vi "QT_DynCall.vi"(0 "QT Ref In":T11, 1 "Frame Grabber Settings":T15={"Name"="", "Digitizer"=0, "Input"=0, "Witdh"=0, "Height"=0, "Input format"=enum."PAL", "Frame rate"=0.0, "Reserved"=0, "Dialogs"=0} {"Frame rate" format="%#1_6g"; "Dialogs" format="%.0b"}, 3 "Compression Settings":T14 {"Dialogs" format="%.0b"; "Comp. Quality" format="%.0x"; "Codec" format="%.0x"}, 4 "Movie Settings":T10 {"Dialogs" format="%.0b"}, 5 "Image in":T5 {"Dialogs" format="%.0b"}, 6 "Sound in":T4 {"Rate" format="%x"}, 7 "error in (no error)":errorcluster, 8 "Selector":T16=enum."Get QT & CIN info", 9 "Video Settings in":T3={"Color format"=1, "Hue"=0.0, "Saturation"=0.0, "Brightness"=0.0, "Contrast"=0.0, "Sharpness"=0.0, "Black Level"=0.0, "White Level"=0.0, "Options"=0, "Dialogs"=0} {"Dialogs" format="%.0b"; "Color format" items=["Black & White (8 bits)", "RGB (24 bits)", "RGBx (32 bits)", "RGBA (32bits)", "RGB B&W (32 bits)", "HSI (24 bits)", "HSIx (32 bits)", "HSI B&W (32 bits)"]; "Brightness" format="%.2f"; "Contrast" format="%.2f"; "Sharpness" format="%.2f"; "Black Level" format="%.2f"; "White Level" format="%.2f"; "Saturation" format="%.2f"; "Hue" format="%.2f"}, 12 "Private":T6={"reserved 1"=4, "reserved 2"=0, "reserved 3"=0, "reserved 4"=0}, 13 "Effect":T9 {"Matrix" format="%.2f"}, 15 "File Settings":T13 {"Dialogs" format="%.0b"}) -> (16 "Info Out":T12, 17 "Video Settings out":T3={"Color format"=1, "Hue"=0.0, "Saturation"=0.0, "Brightness"=0.0, "Contrast"=0.0, "Sharpness"=0.0, "Black Level"=0.0, "White Level"=0.0, "Options"=0, "Dialogs"=0} {"Dialogs" format="%.0b"; "Color format" items=["Black & White (8 bits)", "RGB (24 bits)", "RGBx (32 bits)", "RGBA (32bits)", "RGB B&W (32 bits)", "HSI (24 bits)", "HSIx (32 bits)", "HSI B&W (32 bits)"]; "Brightness" format="%.2f"; "Contrast" format="%.2f"; "Sharpness" format="%.2f"; "Black Level" format="%.2f"; "White Level" format="%.2f"; "Saturation" format="%.2f"; "Hue" format="%.2f"}, 20 "QT Ref Out":T11, 23 "Movie info":T7 {"Tracks"."Rate" format="%.2f"}, 24 "QT Info":T1 {"Digitizers"."In Flags" format="%.0b"; "Digitizers"."Out Flags" format="%.0b"; "Digitizers"."Inputs" items=["Composite", "S-Video", "RGB", "RGB Synch", "YUV", "YUV Synch", "TV Tuner", "sdiln"]; "CIN rev ID" format="%.2f"}, 25 "Image/Movie Out":T5 {"Dialogs" format="%.0b"}, 26 "Sound out":T4 {"Rate" format="%x"}, 27 "error out":errorcluster={"status"=TRUE, "code"=-43, "source"=""})   [LabVIEW 2009]
uses:
  QT_Selector.ctl
  QT_FrameGrabber.ctl
  QT_Video.ctl
  QT_Compression.ctl
  QT_File.ctl
  QT_ErrInfo.ctl
  QT_Image.ctl
  QT_Ref.ctl
  QT_Movie.ctl
  QT_Effect.ctl
  QT_MovieInfo.ctl
  QT_Track.ctl
  QT_Private.ctl
  QT_Sound.ctl
  QT_Info.ctl
  QT_Digitizer.ctl
panel:
  in  "type specifier VI Refnum (for type only)":refnum<vi>
  # "[0,0] [0,1]  [0,2] [1,0].. [2,2]"
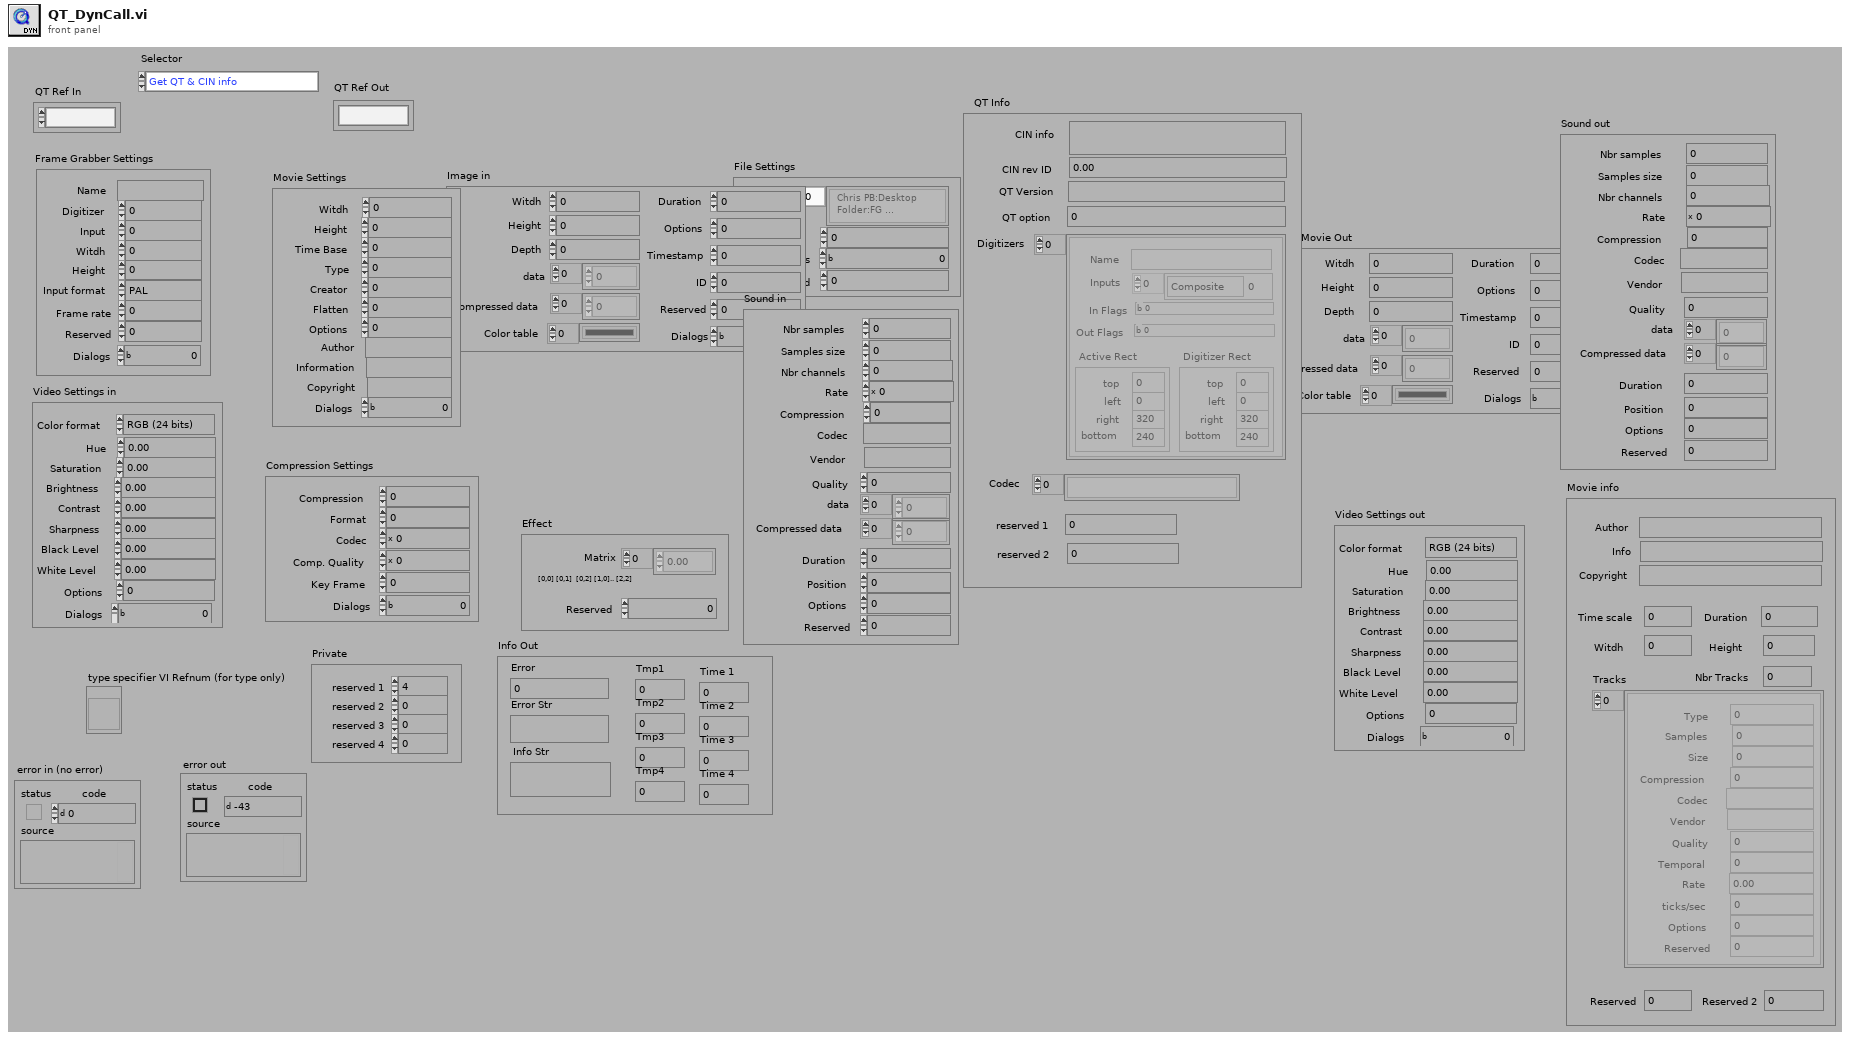
[diagram p1: front panel]
types:
  T1 = typedef "QT_Info.ctl" = cluster{"CIN info":string, "CIN rev ID":dbl, "QT Version":string, "QT option":i32, "Digitizers\n":T2[], "Codec":string[], "reserved 1":i32, "reserved 2":i32}
  T2 = typedef "QT_Digitizer.ctl" = cluster{"Name":string, "Inputs":i32[], "In Flags":i32, "Out Flags":i32, "Digitizer Rect":cluster{"top":i32, "left":i32, "right":i32, "bottom":i32}, "Active Rect":cluster{"top":i32, "left":i32, "right":i32, "bottom":i32}}
  T3 = typedef "QT_Video.ctl" = cluster{"Color format":u32, "Hue":dbl, "Saturation":dbl, "Brightness":dbl, "Contrast":dbl, "Sharpness":dbl, "Black Level":dbl, "White Level":dbl, "Options":i32, "Dialogs":u32}
  T4 = typedef "QT_Sound.ctl" = cluster{"Nbr samples":i32, "Samples size":i32, "Nbr channels":i32, "Rate ":i32, "Compression":i32, "Codec":string, "Vendor":string, "Quality":i32, "data":i16[], "Compressed data":u8[], "Duration":i32, "Position":i32, "Options":i32, "Reserved":i32}
  T5 = typedef "QT_Image.ctl" = cluster{"Witdh":i32, "Height":i32, "Depth":i32, "data":u8[], "Compressed data":u8[], "Color table":u32[], "Duration":i32, "Options":i32, "Timestamp":i32, "ID":i32, "Reserved":i32, "Dialogs":u32}
  T6 = typedef "QT_Private.ctl" = cluster{"reserved 1":i32, "reserved 2":i32, "reserved 3":i32, "reserved 4":i32}
  T7 = typedef "QT_MovieInfo.ctl" = cluster{"Author":string, "Info":string, "Copyright":string, "Time scale":i32, "Duration":i32, "Witdh":i32, "Height":i32, "Nbr Tracks":i32, "Tracks":T8[], "Reserved":i32, "Reserved 2":i32}
  T8 = typedef "QT_Track.ctl" = cluster{"Type":i32, "Samples":i32, "Size":i32, "Compression":i32, "Codec":string, "Vendor":string, "Quality":i32, "Temporal":i32, "Rate ":dbl, "ticks/sec":i32, "Options":i32, "Reserved":i32}
  T9 = typedef "QT_Effect.ctl" = cluster{"Reserved":i32, "Matrix":dbl[]}
  T10 = typedef "QT_Movie.ctl" = cluster{"Witdh":i32, "Height":i32, "Time Base":i32, "Type":i32, "Creator":i32, "Flatten":i32, "Options":i32, "Author":string, "Information":string, "Copyright":string, "Dialogs":u32}
  T11 = typedef "QT_Ref.ctl" = refnum<k1>
  T12 = typedef "QT_ErrInfo.ctl" = cluster{"Error":i32, "Error Str":string, "Info Str":string, "Tmp1":i32, "Tmp2":i32, "Tmp3":i32, "Tmp4":i32, "Time 1":i32, "Time 2":i32, "Time 3":i32, "Time 4":i32}
  T13 = typedef "QT_File.ctl" = cluster{"Paths":string[], "Options":i32, "Dialogs":u32, "Reserved":i32}
  T14 = typedef "QT_Compression.ctl" = cluster{"Compression":i32, "Format":i32, "Codec":i32, "Comp. Quality":i32, "Key Frame":i32, "Dialogs":u32}
  T15 = typedef "QT_FrameGrabber.ctl" = cluster{"Name":string, "Digitizer":i32, "Input":i32, "Witdh":i32, "Height":i32, "Input format":enum32{"NTSC", "PAL", "Secam"}, "Frame rate":dbl, "Reserved":i32, "Dialogs":u32}
  T16 = typedef "QT_Selector.ctl" = enum32{"do nothing", "Get all Sources", "Get Source info", "Open Image", "Save Image to File", "Effect", "Close", "SG Grab", "Compress in Memory", "Decompress to Memory", "New Movie", "Open Movie", "Add Frame", "Get Frame", "Close Movie", "Get QT & CIN info", "SG init", "SG Close", "Open sound file", "Close sound file", "Read sound data", "Write sound data", "Import sound", "Export sound", "Add sound to movie", "Get sound from movie", "reserved", "reserved 1", "reserved 2"}
  T17 = enum32{"invalid CPU target", "Motorola 68K", "PowerPC", "Intel x86", "SPARC", "PA-RISC", "MIPS", "Alpha"}
  T18 = enum32{"invalid OS target", "Mac OS", "Windows 3.1", "Windows 95/NT", "Solaris 1", "Solaris 2", "HP-UX", "PowerMAX", "Linux", "Irix", "Rhapsody", "BeOS", "AIX", "OSF1", "VxWorks", "PharLap", "Carbon", "RTX", "Windows x64", "Linux x64"}
  T19 = enum32{"invalid CPU target", "Motorola 68K", "PowerPC", "Intel x86", "SPARC", "PA-RISC", "MIPS", "Alpha", "ARM", "AMD/Intel x64"}
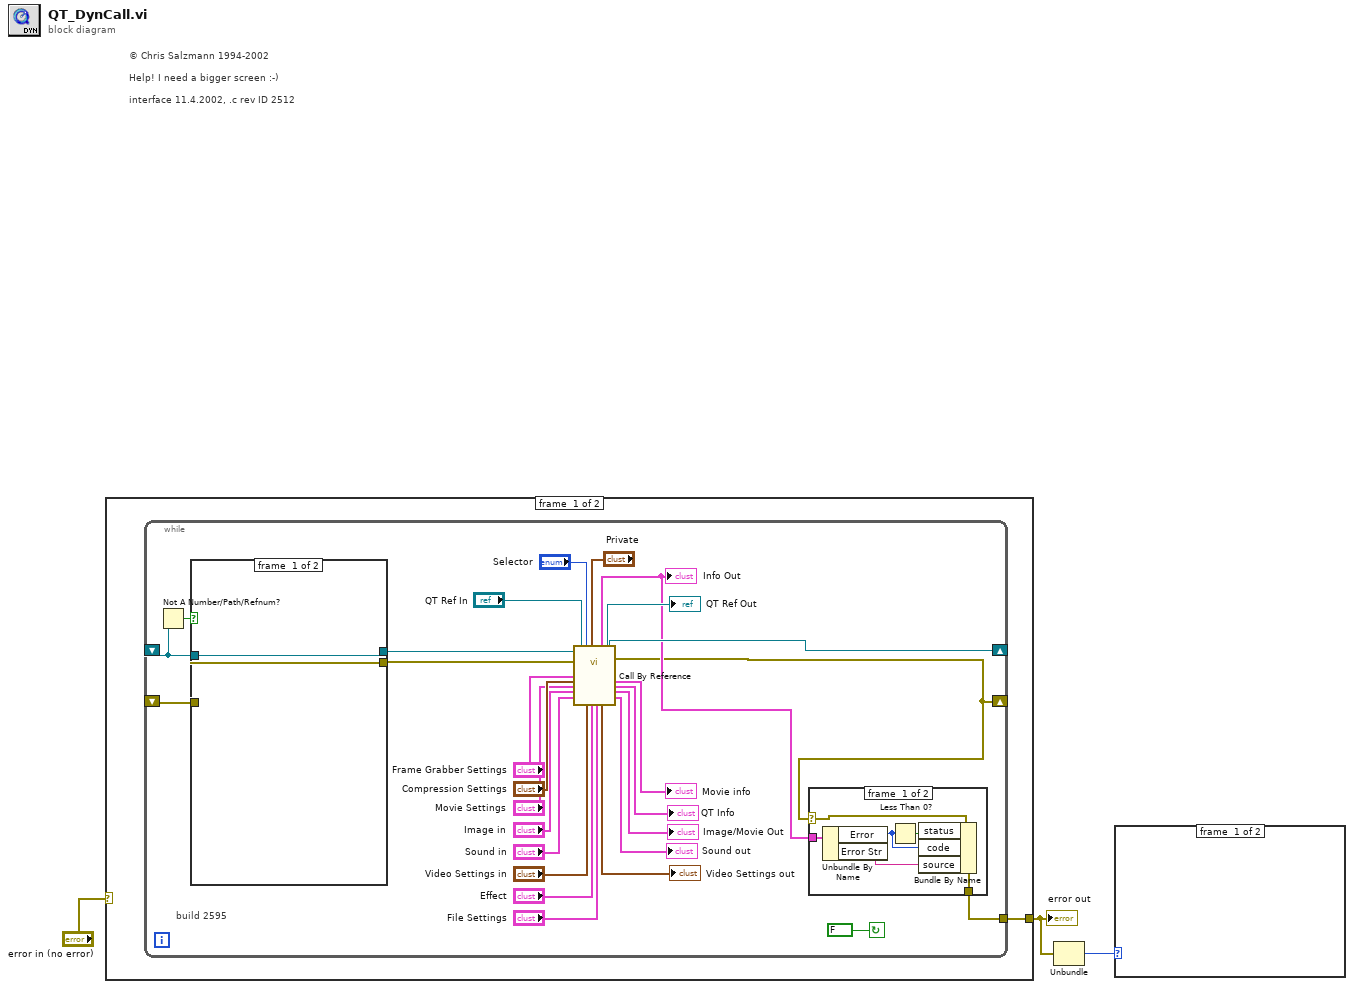
[diagram p0: block diagram]
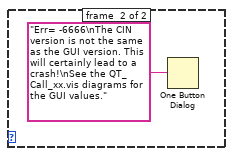
[diagram p2: hidden frame]
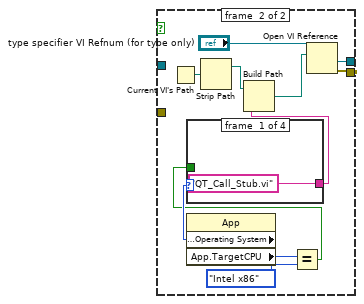
[diagram p4: hidden frame]
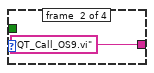
[diagram p5: hidden frame]
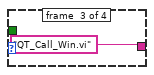
[diagram p6: hidden frame]
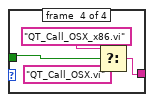
[diagram p7: hidden frame]
diagram:
  # "© Chris Salzmann 1994-2002\n\nHelp! I need a bigger screen :-)\n\ninterface 11.4.2002, .c rev ID 2512"
  n1 = case shown="No Error" "error in (no error)" {
    selector: "error in (no error)" -> [_ w59]
    tunnel: [w4 w59] -> w2
    frame #0 {
      n2 = while {
        tunnel: [w9] -> w4
        shift-left: _ -> [w29]
        shift-right: [w6] -> _
        shift-left: _ -> [w7]
        shift-right: [w28] -> _
        stop <- FALSE continue-if-true
        # "build 2595"
        n3 = Not A Number/Path/Refnum?(number/path/refnum=w7) -> (NaN/Path/Refnum?=w8:bool)
        n4 = case shown="True" w8 {
          tunnel: [w39 w48] -> w30
          tunnel: [w40 w47] -> w5
          tunnel: w29 -> [w39 _]
          tunnel: w7 -> [w40 _]
          frame #0 {
          }
          frame #1 {
            n5 = Current VI's Path() -> (path=w51:path)
            n6 = property class="App"() -> ("Application:Target:Operating System"=w46:T18, "App.TargetCPU"=w43:T19)  [unwired: 2 in, 2 out]
            n7 = Strip Path(path=w51) -> (stripped path=w50:path)  [unwired: 1 out]
            n8 = Equal?(x=w43, y=T17."Intel x86") -> (x = y?=w41:bool)
            n9 = case shown="\"Carbon\"" w46 {
              tunnel: ["QT_Call_Stub.vi" ("name or relative path") "QT_Call_OS9.vi" ("name or relative path") "QT_Call_Win.vi" ("name or relative path") w56] -> w45
              tunnel: w41 -> [_ _ _ w55]
              frame #0 {
              }
              frame #1 {
              }
              frame #2 {
              }
              frame #3 {
                n10 = Select(t="QT_Call_OSX_x86.vi" ("name or relative path"), s=w55, f="QT_Call_OSX.vi" ("name or relative path")) -> (s? t:f=w56:string)
              }
            }
            n11 = Build Path(base path=w50, name or relative path=w45) -> (appended path=w49:path)
            n12 = Open VI Reference(type specifier VI Refnum (for type only)="type specifier VI Refnum (for type only)", vi path=w49) -> (vi reference=w47:refnum<vi>, error out=w48:errorcluster)  [unwired: 1 in, 3 out]
          }
        }
        n13 = call-by-ref "?"(reference=w5, error in=w30, "QT Ref In"="QT Ref In", "Frame Grabber Settings"="Frame Grabber Settings", "Compression Settings"="Compression Settings", "Movie Settings"="Movie Settings", "Image in"="Image in", "Sound in"="Sound in", "Selector"="Selector", "Video Settings in"="Video Settings in", "Private"="Private", "Effect"="Effect", "File Settings"="File Settings") -> (reference out=w28:refnum<vi>, error out=w6:errorcluster, "Info Out"=w25:T12, "Video Settings out"=→"Video Settings out":T3, "QT Ref Out"=→"QT Ref Out":T11, "Movie info"=→"Movie info":T7, "QT Info"=→"QT Info":T1, "Image/Movie Out"=→"Image/Movie Out":T5, "Sound out"=→"Sound out":T4)  [unwired: 2 in]
        "Info Out" <- w25
        n14 = case shown="No Error" w6 {
          selector: w6 -> [w36 w38]
          tunnel: [w32 w38] -> w9
          tunnel: w25 -> [w37 _]
          frame #0 {
            n15 = Unbundle By Name(w37) -> ("Error"=w34:i32, "Error Str"=w33:string)
            n16 = Less Than 0?(x=w34) -> (x < 0?=w35:bool)
            n17 = Bundle By Name(cluster=w36, "status"=w35, "code"=w34, "source"=w33) -> (w32:errorcluster)
          }
          frame #1 {
          }
        }
      }
    }
    frame #1 {
    }
  }
  "error out" <- w2
  n18 = Unbundle(w2) -> ("code"=w1:i32)  [unwired: 2 out]
  n19 = case shown="-6666" w1 {
    frame #0 {
    }
    frame #1 {
      n20 = One Button Dialog(message="Err= -6666\nThe CIN version is not the same as the GUI version. This will certainly lead to a crash!\nSee the QT_Call_xx.vis diagrams for the GUI values.") -> ()  [unwired: 2 out]
    }
  }
